vi "AutoPowerMesa 2.vi"() -> ()   [LabVIEW 2015]
panel:
  in  "Mode02 2":bool
  in  "Mode02":bool
  out "ok? 2":bool
  out "ok?":bool
  out "EOff":string
  out "EOn":string
  out "IOff":string
  out "IOn":string
  in  "VISA resource name":refnum<visa-resource-name>="COM11"
  in  "EnOff":bool
  in  "EnOn":bool
  in  "IgnOff":bool
  in  "IgnOn":bool
  in  "stop":bool
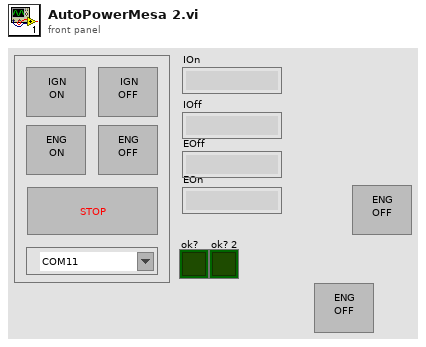
[diagram p1: front panel]
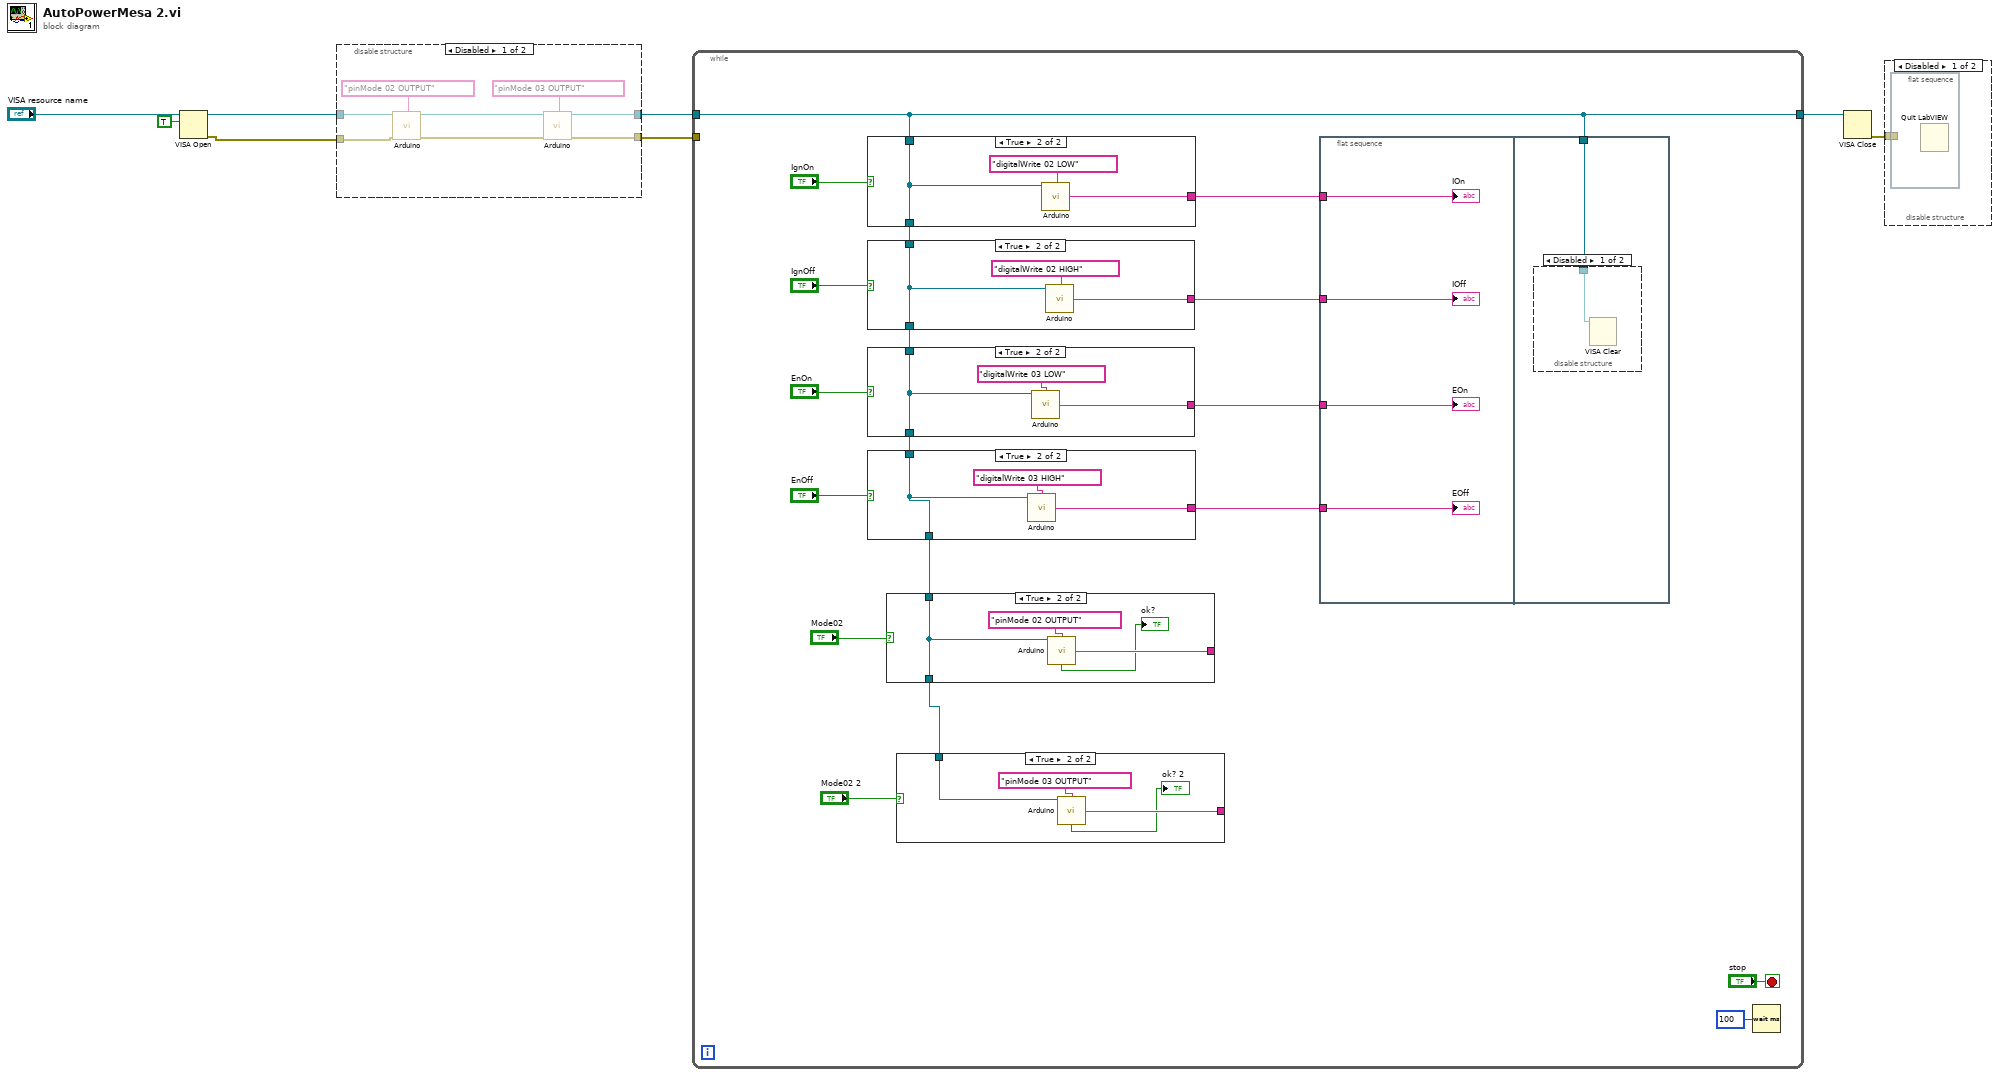
[diagram p0: block diagram]
diagram:
  n1 = VISA Open(duplicate session (F)=TRUE, VISA resource name="VISA resource name") -> (VISA resource name=w4:refnum<visa-resource-name>, error out=w1:errorcluster)  [unwired: 3 in]
  n2 = disable-structure shown="Disabled" {
    disable-tunnel: w4 -> [w18 w20]
    disable-tunnel: [w13 w20] -> w3
    disable-tunnel: [w12 w19] -> w2
    disable-tunnel: w1 -> [w9 w19]
    frame Disabled {
      n3 = call "Arduino.vi"("Serial Com"=w18, "Function"="pinMode 02 OUTPUT", "error in (no error)"=w9) -> ("Serial Out"=w14:refnum<visa-resource-name>, "ok?"=w11:bool, "error out"=w15:errorcluster)  [unwired: 9 in, 1 out]
      n4 = call "Arduino.vi"("Serial Com"=w14, "Function"="pinMode 03 OUTPUT", "error in (no error)"=w15) -> ("Serial Out"=w13:refnum<visa-resource-name>, "ok?"=w10:bool, "error out"=w12:errorcluster)  [unwired: 9 in, 1 out]
    }
    frame Enabled {
    }
  }
  n5 = while {
    tunnel: w3 -> [w25]
    tunnel: [w25] -> w8
    tunnel: w2 -> [_]
    stop <- "stop" stop-if-true
    n6 = case shown="True" "IgnOn" {
      tunnel: w25 -> [w66 w67]
      tunnel: [w66 w67] -> w36
      tunnel: [_ w68] -> w29
      frame False {
      }
      frame True {
        n7 = call "Arduino.vi"("Serial Com"=w67, "Function"="digitalWrite 02 LOW") -> ("result"=w68:string)  [unwired: 10 in, 3 out]
      }
    }
    n8 = case shown="True" "IgnOff" {
      tunnel: w36 -> [w62 w63]
      tunnel: [w62 w63] -> w33
      tunnel: [_ w65] -> w28
      frame False {
      }
      frame True {
        n9 = call "Arduino.vi"("Serial Com"=w63, "Function"="digitalWrite 02 HIGH") -> ("result"=w65:string)  [unwired: 10 in, 3 out]
      }
    }
    n10 = case shown="True" "EnOn" {
      tunnel: w33 -> [w58 w61]
      tunnel: [w58 w61] -> w34
      tunnel: [_ w59] -> w27
      frame False {
      }
      frame True {
        n11 = call "Arduino.vi"("Serial Com"=w61, "Function"="digitalWrite 03 LOW") -> ("result"=w59:string)  [unwired: 10 in, 3 out]
      }
    }
    n12 = case shown="True" "EnOff" {
      tunnel: w34 -> [w54 w55]
      tunnel: [_ w56] -> w26
      tunnel: [w54 w55] -> w23
      frame False {
      }
      frame True {
        n13 = call "Arduino.vi"("Serial Com"=w55, "Function"="digitalWrite 03 HIGH") -> ("result"=w56:string)  [unwired: 10 in, 3 out]
      }
    }
    n14 = case shown="True" "Mode02" {
      tunnel: w23 -> [w43 w45]
      tunnel: [_ w46] -> _
      tunnel: [w43 w45] -> w21
      frame False {
      }
      frame True {
        n15 = call "Arduino.vi"("Serial Com"=w45, "Function"="pinMode 02 OUTPUT") -> ("result"=w46:string, "ok?"=→"ok?":bool)  [unwired: 10 in, 2 out]
      }
    }
    n16 = case shown="True" "Mode02 2" {
      tunnel: w21 -> [_ w41]
      tunnel: [_ w40] -> _
      frame False {
      }
      frame True {
        n17 = call "Arduino.vi"("Serial Com"=w41, "Function"="pinMode 03 OUTPUT") -> ("result"=w40:string, "ok?"=→"ok? 2":bool)  [unwired: 10 in, 2 out]
      }
    }
    n18 = flat-sequence {
      tunnel: w29 -> [w51]
      tunnel: w28 -> [w50]
      tunnel: w27 -> [w49]
      tunnel: w26 -> [w48]
      tunnel: w25 -> [w52]
      frame #0 {
        "IOn" <- w51
        "IOff" <- w50
        "EOn" <- w49
        "EOff" <- w48
      }
      frame #1 {
        n19 = disable-structure shown="Disabled" {
          disable-tunnel: w52 -> [w53 _]
          frame Disabled {
            n20 = VISA Clear(VISA resource name=w53) -> ()  [unwired: 1 in, 2 out]
          }
          frame Enabled {
          }
        }
      }
    }
    n21 = Wait (ms)(milliseconds to wait=u32 100) -> ()  [unwired: 1 out]
  }
  n22 = VISA Close(VISA resource name=w8) -> (error out=w7:errorcluster)  [unwired: 1 in]
  n23 = disable-structure shown="Disabled" {
    disable-tunnel: w7 -> [w70 _]
    frame Disabled {
      n24 = flat-sequence {
        tunnel: w70 -> [_]
        frame #0 {
          n25 = Quit LabVIEW() -> ()  [unwired: 1 in]
        }
      }
    }
    frame Enabled {
    }
  }
